vi "Calibration High Limit (Read).vi"(6 "ISOBUS address":T3=-1 caption="ISOBUS address (-1)", 8 "error in":errorcluster, 11 "Mercury Reference In":T4) -> (0 "error out":errorcluster, 1 "Unit":T1, 2 "Hot Limit":dbl, 3 "Mercury Reference Out":T4, 4 "Valid?":T2)   [LabVIEW 2015, in "Mercury iXX.lvlib" / "Pressure.lvlib"]
doc: "Read the current hot limit of the selected pressure device."
uses:
  Pressure.lvlib
  Controls/Mercury Reference.ctl
  Controls/Comms Transport Layer.ctl
  Private/Controls/Query Dynamic Reference.ctl
  Controls/ISOBus Address.ctl
  Controls/Is Valid LED.ctl
  Controls/Unit String.ctl
  Private/Controls/Command Verbs.ctl
  Mercury iXX.lvlib
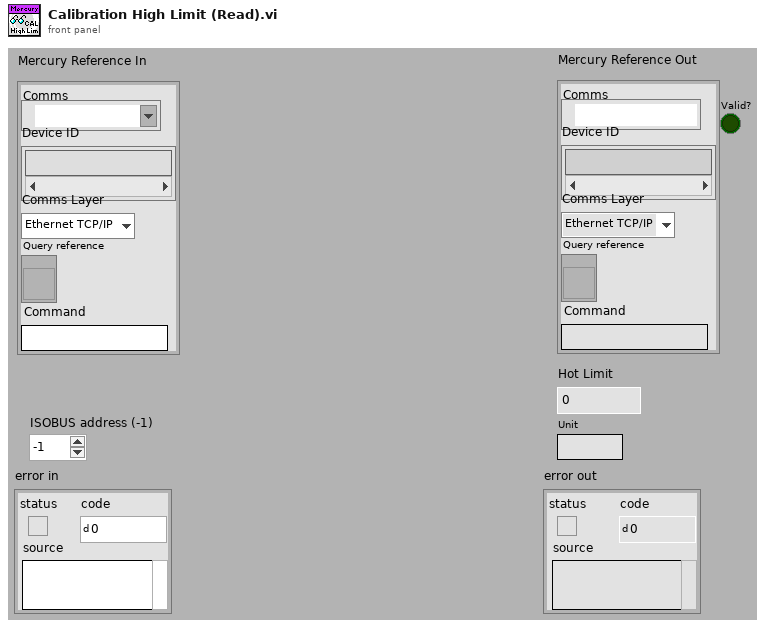
[diagram p1: front panel]
types:
  T1 = typedef "Mercury iXX.lvlib/Unit String.ctl" = string
  T2 = typedef "Mercury iXX.lvlib/Is Valid LED.ctl" = bool
  T3 = typedef "Mercury iXX.lvlib/ISOBus Address.ctl" = i32
  T4 = typedef "Mercury iXX.lvlib/Mercury Reference.ctl" = cluster{"Comms":refnum<visa-resource-name>, "Device ID":string[], "Comms Layer":T5, "Command":string, "Query reference":T6}
  T5 = typedef "Mercury iXX.lvlib/Comms Transport Layer.ctl" = enum16{"Ethernet TCP/IP", "USB", "ISOBus - RS-232", "GPIB"}
  T6 = typedef "Mercury iXX.lvlib/Query Dynamic Reference.ctl" = refnum<vi>
  T7 = typedef "Mercury iXX.lvlib/Command Verbs.ctl" = string
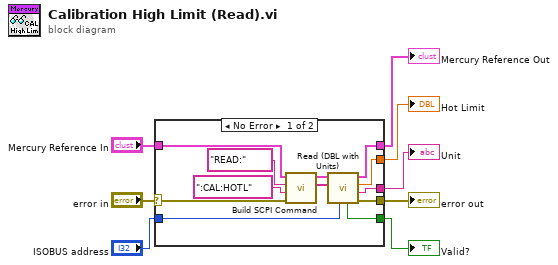
[diagram p0: block diagram]
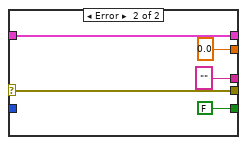
[diagram p2: hidden frame]
diagram:
  n1 = case shown="No Error" "error in" {
    selector: "error in" -> [w9 w25]
    tunnel: "Mercury Reference In" -> [w16 w24]
    tunnel: [w15 w24] -> w7
    tunnel: [w14 w25] -> w6
    tunnel: "ISOBUS address" -> [w13 _]
    tunnel: [w12 T2 FALSE ("Valid?")] -> w4
    tunnel: [w11 0.0 ("Data (Dbl)")] -> w3
    tunnel: [w10 T1 "" ("Unit")] -> w2
    frame No Error {
      n2 = call "Build SCPI Command.vi"("error in"=w9, "Noun(s)"=":CAL:HOTL" ("Command"), "Verb"=T7 "READ:", "Mercury Reference In"=w16) -> ("SCPI Message(s)"=w19:string[], "Mercury Reference Out"=w20:T4)  [unwired: 6 out]
      n3 = call "Read (DBL with Units).vi"("ISOBUS address"=w13, "SCPI Message(s)"=w19, "Mercury Reference In"=w20) -> ("error out"=w14:errorcluster, "Unit"=w10:T1, "Data (Dbl)"=w11:dbl, "Mercury Reference Out"=w15:T4, "Valid?"=w12:T2)  [unwired: 1 in, 3 out]
    }
    frame Error {
    }
  }
  "Mercury Reference Out" <- w7
  "error out" <- w6
  "Hot Limit" <- w3
  "Valid?" <- w4
  "Unit" <- w2
